vi "HP 4285A impedance read.vi"() -> ()   [LabVIEW 2009]
uses:
  <instrlib>/Agilent 428X Series/Agilent 428X Series.lvlib
panel:
  out "phase (degrees)":dbl
  out "Z (ohms)":dbl
  in  "Frequency Value (Hz)":dbl=1000000.0 min=20.0 max=30000000.0 step=1.0 format="%.4e"
  in  "stop":bool
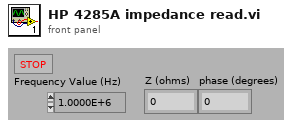
[diagram p1: front panel]
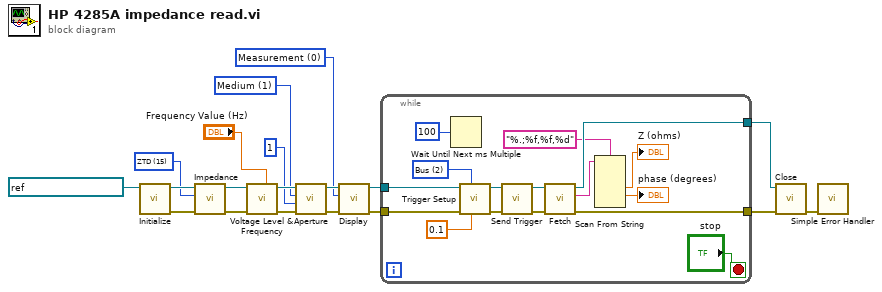
[diagram p0: block diagram]
diagram:
  w3 = u32 0 items=["Measurement", "Bin Number", "Bin Count", "List", "Measurement Setup", "Correction Setup", "Limit Table", "List Setup", "System", "Catalog", "SelfTest", "Line String"] ("Display Page (0: Measurement)")
  w7 = u32 1 items=["Short", "Medium", "Long"] ("Integ Time (0: Short)")
  w9 = u32 15 items=["CPD", "CPQ", "CPG", "CPRP", "CSD", "CSQ", "CSRS", "LPQ", "LPD", "LPG", "LPRP", "LSD", "LSQ", "LSRS", "RX", "ZTD", "ZTR", "GB", "YTD", "YTR"] ("Imp Type (0: CPD)")
  n1 = call <instrlib>:"Initialize.vi"("VISA resource name"=refnum<visa-resource-name> "GPIB0::19::INSTR") -> ("error out"=w15:errorcluster, "VISA resource name out"=w17:refnum<visa-resource-name>)  [unwired: 9 in]
  n2 = call <instrlib>:"Impedance.vi"("error in (no error)"=w15, "Imp Type (0: CPD)"=w9, "VISA resource name"=w17) -> ("error out"=w14:errorcluster, "VISA resource name out"=w18:refnum<visa-resource-name>)  [unwired: 7 in]
  n3 = call <instrlib>:"Voltage Level & Frequency.vi"("Frequency Value (20.0 Hz)"="Frequency Value (Hz)", "error in (no error)"=w14, "VISA resource name"=w18) -> ("error out"=w13:errorcluster, "VISA resource name out"=w19:refnum<visa-resource-name>)  [unwired: 7 in]
  n4 = call <instrlib>:"Aperture.vi"("error in (no error)"=w13, "Averaging Rate (1)"=i16 1, "Integ Time (0: Short)"=w7, "VISA resource name"=w19) -> ("error out"=w4:errorcluster, "VISA resource name out"=w5:refnum<visa-resource-name>)  [unwired: 6 in]
  n5 = call <instrlib>:"Display.vi"("error in (no error)"=w4, "Display Page (0: Measurement)"=w3, "VISA resource name"=w5) -> ("error out"=w1:errorcluster, "VISA resource name out"=w2:refnum<visa-resource-name>)  [unwired: 7 in]
  n6 = while {
    tunnel: [w33] -> w12
    tunnel: [w34] -> w10
    tunnel: w2 -> [w21]
    tunnel: w1 -> [w20]
    stop <- "stop" stop-if-true
    w27 = u32 2 items=["Internal", "External", "Bus", "Hold"] ("Trigger Source (0: Internal)")
    n7 = Wait Until Next ms Multiple(millisecond multiple=u32 100) -> ()  [unwired: 1 out]
    n8 = call <instrlib>:"Trigger Setup.vi"("Delay Value (s) (0.0)"=0.1, "Trigger Source (0: Internal)"=w27, "error in (no error)"=w20, "VISA resource name"=w21) -> ("error out"=w26:errorcluster, "VISA resource name out"=w25:refnum<visa-resource-name>)  [unwired: 6 in]
    n9 = call <instrlib>:"Send Trigger.vi"("error in (no error)"=w26, "VISA resource name"=w25) -> ("error out"=w23:errorcluster, "VISA resource name out"=w24:refnum<visa-resource-name>)  [unwired: 8 in]
    n10 = call <instrlib>:"Fetch.vi"("error in (no error)"=w23, "VISA resource name"=w24) -> ("error out"=w33:errorcluster, "Returned Data"=w32:string, "VISA resource name out"=w34:refnum<visa-resource-name>)  [unwired: 7 in]
    n11 = Scan From String(format string="%.;%f,%f,%d", input string=w32) -> (output 1=→"Z (ohms)":dbl, output 2=→"phase (degrees)":dbl)  [unwired: 6 in, 3 out]
  }
  n12 = call <instrlib>:"Close.vi"("error in (no error)"=w12, "VISA resource name"=w10) -> ("error out"=w11:errorcluster)  [unwired: 9 in]
  n13 = call <vilib>:"Simple Error Handler.vi"("error in (no error)"=w11) -> ()  [unwired: 4 in, 5 out]
